vi "usbsimplecommand.vi"() -> ()   [LabVIEW 2022 SP3]
uses:
  <vilib>/Instr/_visa.llb/VISA Configure Serial Port (Instr).vi
panel:
  in  "write buffer":string
  out "read buffer":string
  in  "VISA resource name":refnum<visa-resource-name>
  # "This VI example can send any command to Numato Lab's USB GPIO or USB Relay products. Please follow the steps below to send a command and view the response. The response is not parsed and displayed raw."
  # "1. Select a COM port below"
  # "2. Type the command below"
  # "3. Press the run button on Frontpanel toolbar"
  # "4. Result will be displayed below"
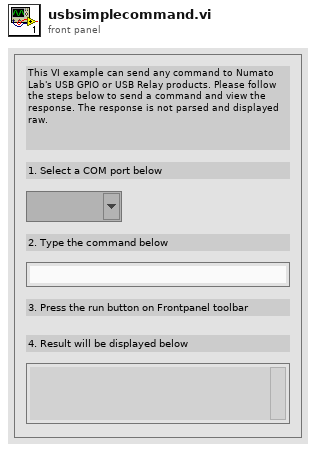
[diagram p1: front panel]
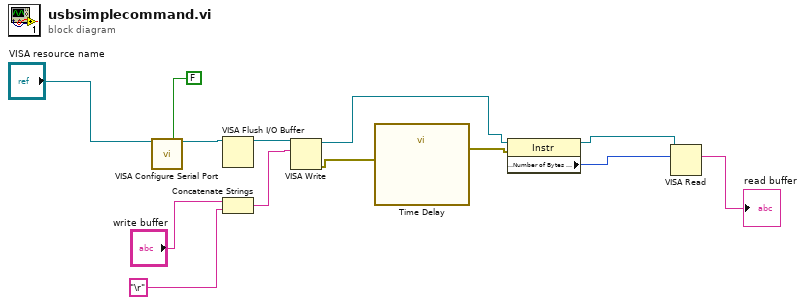
[diagram p0: block diagram]
diagram:
  n1 = call-poly "VISA Configure Serial Port"("VISA resource name"="VISA resource name", "Enable Termination\nChar (T)"=FALSE ("Enable Termination\nChar (T)")) -> ("VISA resource name out"=w8:refnum<visa-resource-name>)  [unwired: 12 in, 1 out]
  n2 = VISA Flush I/O Buffer(VISA resource name=w8) -> (VISA resource name out=w7:refnum<visa-resource-name>)  [unwired: 2 in, 1 out]
  n3 = Concatenate Strings("write buffer", "\r") -> (w3:string)
  n4 = VISA Write(VISA resource name=w7, write buffer=w3) -> (VISA resource name out=w4:refnum<visa-resource-name>, error out=w6:errorcluster)  [unwired: 1 in, 1 out]
  n5 = call "Time Delay"("error in (no error)"=w6) -> ("error out"=w5:errorcluster)  [unwired: 10 in]
  n6 = property class="Instr"(reference=w4, error in=w5) -> (reference out=w11:refnum<visa-resource-name>, "Serial Settings:Number of Bytes at Serial Port"=w10:u32)  [unwired: 1 out]
  n7 = VISA Read(VISA resource name=w11, byte count=w10) -> (read buffer=→"read buffer":string)  [unwired: 1 in, 3 out]
